vi "Matches.vi"(8 "error in (no error)":errorcluster, 10 "Actual":variant, 11 "Collection Contains in":refnum<class "Collection Contains.lvclass">) -> (0 "error out":errorcluster, 2 "Result":bool, 3 "Collection Contains out":refnum<class "Collection Contains.lvclass">)   [LabVIEW 2017, in "Transparent Assertions.lvlib" / "Constraints.lvlib" / "Collection Contains.lvclass"]
doc: "Evaluates the constraint for <B>Actual</B>. Returns true if the constraint is met."
uses:
  Collection Contains.lvclass
  Collection Contains.lvclass/Collection Contains.ctl
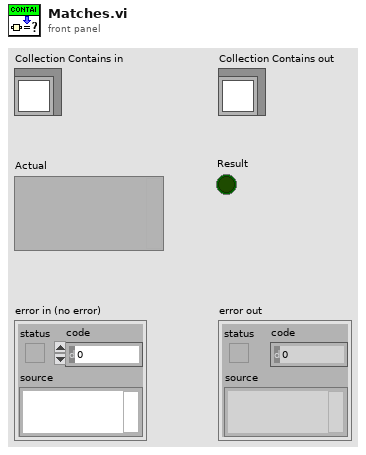
[diagram p1: front panel]
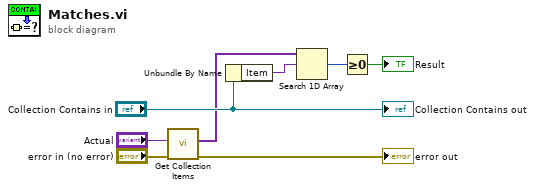
[diagram p0: block diagram]
diagram:
  n1 = call "Get Collection Items.vi"("error in (no error)"="error in (no error)", "Collection"="Actual") -> ("error out"=→"error out":errorcluster, "Items"=w3:variant[])  [unwired: 8 in]
  n2 = Unbundle By Name("Collection Contains in") -> ("Item"=w7:variant)
  n3 = Search 1D Array(1D array=w3, element=w7) -> (index of element=w6:i32)  [unwired: 1 in]
  n4 = Greater Or Equal To 0?(x=w6) -> (x >= 0?=→"Result":bool)
  "Collection Contains out" <- "Collection Contains in"
